vi "Angle Degrees.vi"() -> ()   [LabVIEW 2016]
panel:
  in  "Angle Degrees":dbl
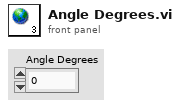
[diagram p1: front panel]
diagram:
